vi "BrakeLoad_SineWaveGenerator.vi"(10 "Max Right Travel":dbl=1.25, 11 "Max Left Travel":dbl=1.25) -> (2 "Load  Curve":dbl[](graph), 3 "Trigger Point & Load Level":dbl[][](array[numeric]) format="%#_3f")   [LabVIEW 2026, in "Acquisition.lvlib"]
uses:
  Acquisition.lvlib
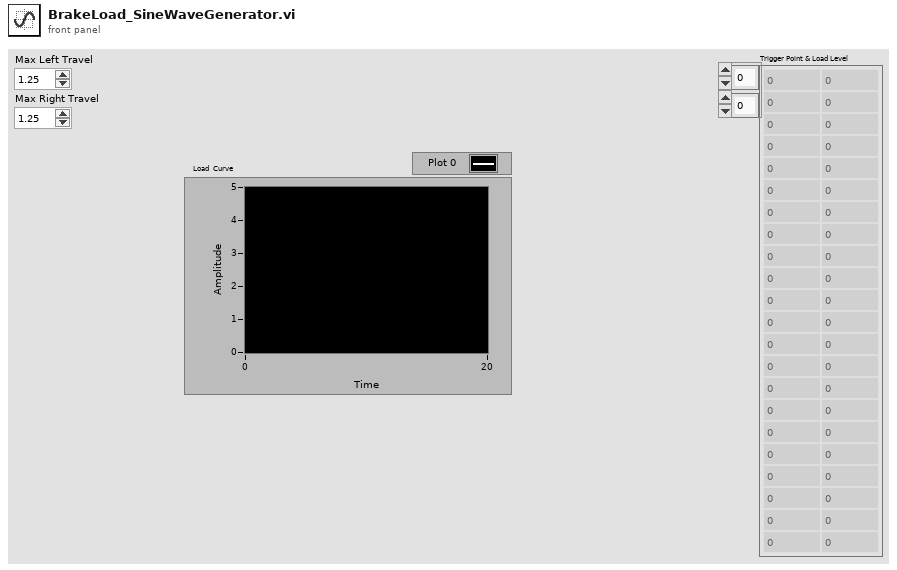
[diagram p1: front panel]
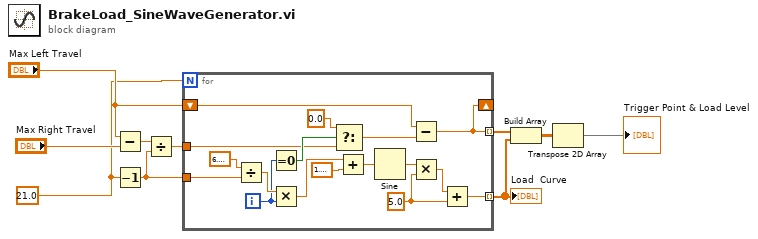
[diagram p0: block diagram]
diagram:
  w3 = 21.0 ("y")
  n1 = Subtract(x="Max Left Travel", y="Max Right Travel") -> (x-y=w9:dbl)
  n2 = Decrement(x=w3) -> (x-1=w2:dbl)
  n3 = Divide(x=w9, y=w2) -> (x/y=w10:dbl)
  n4 = for {
    N: w3 -> [_]
    tunnel: w10 -> [w13]
    shift-right: [w26] -> _
    shift-left: "Max Left Travel" -> [w27]
    tunnel: [w26] -> w8 mode=indexing
    tunnel: [w20] -> w7 mode=indexing
    tunnel: w2 -> [w11]
    i -> [w16]
    w21 = 5.0 ("y")
    n5 = Divide(x=6.283185307179586, y=w11) -> (x/y=w24:dbl)
    n6 = Equal To 0?(x=w16) -> (x = 0?=w14:bool)
    n7 = Multiply(x=w24, y=w16) -> (x*y=w19:dbl)
    n8 = Select(t=0.0, s=w14, f=w13) -> (s? t:f=w15:dbl)
    n9 = Add(x=w19, y=1.5707963267948966) -> (x+y=w18:dbl)
    n10 = Sine(x=w18) -> (sin(x)=w23:dbl)
    n11 = Subtract(x=w27, y=w15) -> (x-y=w26:dbl)
    n12 = Multiply(x=w23, y=w21) -> (x*y=w22:dbl)
    n13 = Add(x=w22, y=w21) -> (x+y=w20:dbl)
  }
  "Load  Curve" <- w7
  n14 = Build Array(w8, w7) -> (w6:dbl[][])
  n15 = Transpose 2D Array(2D array=w6) -> (transposed array=→"Trigger Point & Load Level":dbl[][])
